vi "Get channel metadata.vi"(0 "reference in":refnum<class "TDMS_DataHandler.lvclass">, 2 "channel name":string, 5 "error in (no error)":errorcluster) -> (14 "reference out":refnum<class "TDMS_DataHandler.lvclass">, 16 "Tdms metadata out":T1, 19 "error out":errorcluster)   [LabVIEW 2019, in "TDMS_DataHandler.lvclass"]
uses:
  TDMS_DataHandler.lvclass
  Fcurve Meta data.ctl
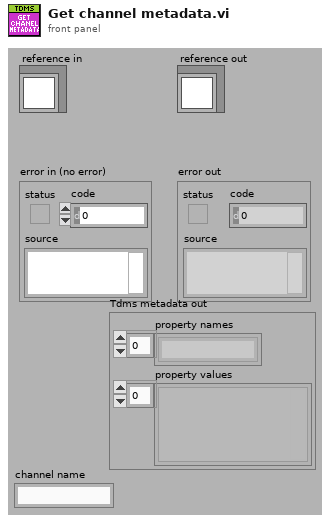
[diagram p1: front panel]
types:
  T1 = cluster{"property names":string[], "property values":variant[]}
  T2 = typedef "TDMS_DataHandler.lvclass/Fcurve Meta data.ctl" = cluster{"property names":string[], "property values":variant[]}
  T3 = typedef "TDMS_DataHandler.lvclass/ObjectAttributesRef.ctl" = refnum<data-value>
  T4 = typedef "TDMS_DataHandler.lvclass/ObjectAttributes.ctl" = cluster{"Directory":path, "FilePath":path, "FileRef":refnum<k34>, "ExperimentName":string, "GroupName":string, "ChannelNames":string[], "Datum":waveform(dbl)[], "Group_Metadata":cluster{"property names":string[], "property values":variant[]}, "Channel_Metadata":cluster{"property names":string[], "property values":variant[]}}
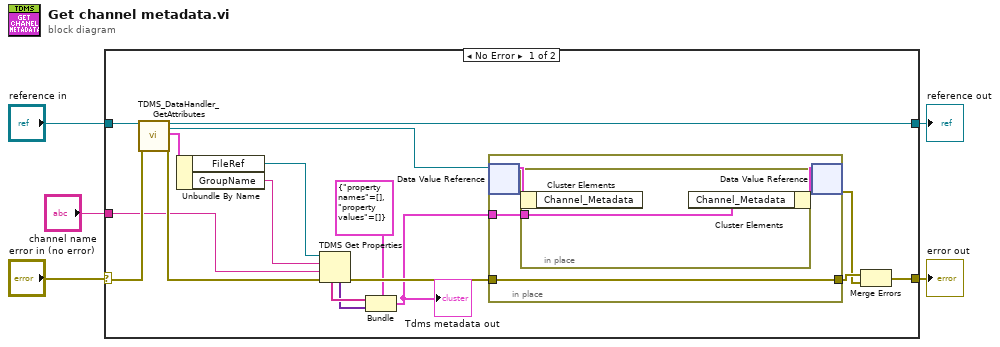
[diagram p0: block diagram]
diagram:
  n1 = case shown="No Error" "error in (no error)" {
    selector: "error in (no error)" -> [w19 w29]
    tunnel: [w22 w29] -> w4
    tunnel: [w20 w28] -> w2
    tunnel: "reference in" -> [w21 w28]
    tunnel: "channel name" -> [w6 _]
    frame No Error {
      n2 = call "TDMS_DataHandler_GetAttributes.vi"("reference in"=w21, "error in (no error)"=w19) -> ("reference out"=w20:refnum<class "TDMS_DataHandler.lvclass">, "attributes ref"=w15:T3, "attributes"=w18:T4, "error out"=w13:errorcluster)  [unwired: 14 in]
      n3 = Unbundle By Name(w18) -> ("FileRef"=w14:refnum<k34>, "GroupName"=w7:string)
      n4 = TDMS Get Properties(8:w13, 9:w6, 10:w7, 11:w14) -> (0:w12:errorcluster, 4:w10:variant[], 6:w11:string[])  [unwired: 2 in, 3 out]
      n5 = Bundle(cluster=T2 {"property names"=[], "property values"=[]} ("Fcurve Metadata"), "property names"=w11, "property values"=w10) -> (w8:T2)
      "Tdms metadata out" <- w8
      n6 = in-place {
        in-place-border: w12 -> [w24]
        in-place-border: [w24] -> w17
        in-place-border: w8 -> [w23]
        n7 = in-place-dvr #1(w15) -> (w25:T4)  [unwired: 1 out]
        n8 = in-place {
          in-place-border: w23 -> [w27]
          n9 = in-place-cluster #2(w25) -> ()  [unwired: 1 out]
          n10 = in-place-cluster #2("Channel_Metadata"=w27) -> (w26:T4)
        }
        n11 = in-place-dvr #1(w26) -> (w16:errorcluster)  [unwired: 1 out]
      }
      n12 = Merge Errors(w17, w16) -> (w22:errorcluster)
    }
    frame Error {
    }
  }
  "error out" <- w4
  "reference out" <- w2
